vi "Set Collector Speed.vi"(10 "Buttons":T1) -> (3 "Collector Speed":dbl)   [LabVIEW 2011]
uses:
  <vilib>/Rock Robotics/WPI/Joystick/WPI_JoystickButtonState.ctl
  Robot Global Data.vi
panel:
  out "number":u32
  in  "Collector Setting":dbl(slide)=0.6 scale=0.0..1.0
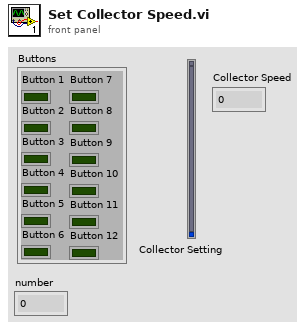
[diagram p1: front panel]
types:
  T1 = typedef "WPI_JoystickButtonState.ctl" = cluster{"Button 1":bool, "Button 2":bool, "Button 3":bool, "Button 4":bool, "Button 5":bool, "Button 6":bool, "Button 7":bool, "Button 8":bool, "Button 9":bool, "Button 10":bool, "Button 11":bool, "Button 12":bool}
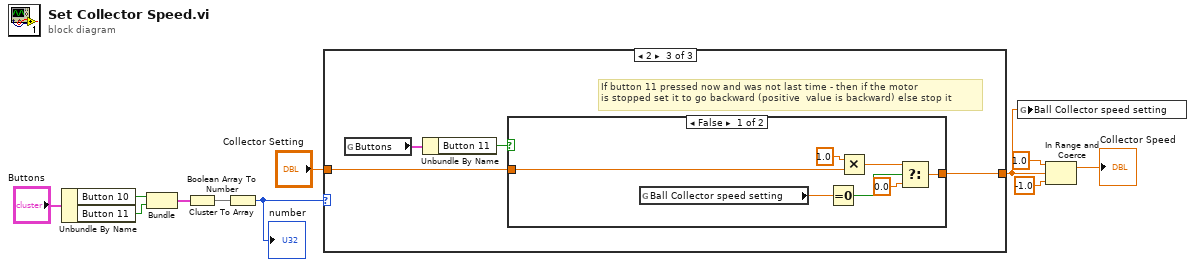
[diagram p0: block diagram]
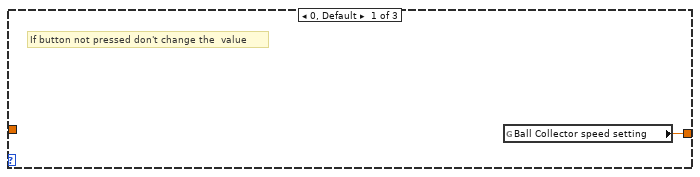
[diagram p2: hidden frame]
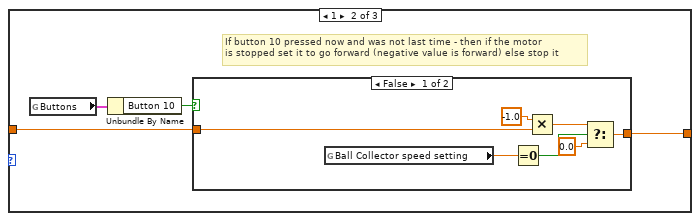
[diagram p3: hidden frame]
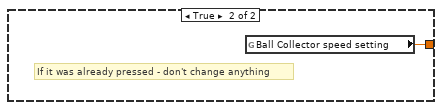
[diagram p4: hidden frame]
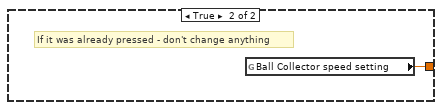
[diagram p5: hidden frame]
diagram:
  n1 = Unbundle By Name("Buttons") -> ("Button 10"=w6:bool, "Button 11"=w5:bool)
  n2 = Bundle("Button 10"=w6, "Button 11"=w5) -> (w4:cluster{"Button 10":bool, "Button 11":bool})  [unwired: 1 in]
  n3 = Cluster To Array(cluster=w4) -> (array=w3:bool[])
  n4 = Boolean Array To Number(Boolean array=w3) -> (number=w2:u32)
  "number" <- w2
  n5 = case shown="2" w2 {
    tunnel: [w12 w14 w26] -> w1
    tunnel: "Collector Setting" -> [_ w13 w25]
    frame 0, Default {
      # "If button not pressed don't change the  value"
      n6 = global read "Robot Global Data.vi" "Ball Collector speed setting"() -> (w12:dbl)
    }
    frame 1 {
      # "If button 10 pressed now and was not last time - then if the motor \nis stopped set it to go forward (negative value is forward) else stop it"
      n7 = global read "Robot Global Data.vi" "Buttons"() -> (w16:T1)
      n8 = Unbundle By Name(w16) -> ("Button 10"=w15:bool)
      n9 = case shown="False" w15 {
        tunnel: [w20 w24] -> w14
        tunnel: w13 -> [w19 _]
        frame False {
          n10 = global read "Robot Global Data.vi" "Ball Collector speed setting"() -> (w22:dbl)
          n11 = Equal To 0?(x=w22) -> (x = 0?=w23:bool)
          n12 = Multiply(x=-1.0, y=w19) -> (x*y=w17:dbl)
          n13 = Select(t=w17, s=w23, f=0.0) -> (s? t:f=w20:dbl)
        }
        frame True {
          # "If it was already pressed - don't change anything"
          n14 = global read "Robot Global Data.vi" "Ball Collector speed setting"() -> (w24:dbl)
        }
      }
    }
    frame 2 {
      # "If button 11 pressed now and was not last time - then if the motor \nis stopped set it to go backward (positive  value is backward) else stop it"
      n15 = global read "Robot Global Data.vi" "Buttons"() -> (w28:T1)
      n16 = Unbundle By Name(w28) -> ("Button 11"=w27:bool)
      n17 = case shown="False" w27 {
        tunnel: [w32 w36] -> w26
        tunnel: w25 -> [w31 _]
        frame False {
          n18 = global read "Robot Global Data.vi" "Ball Collector speed setting"() -> (w34:dbl)
          n19 = Equal To 0?(x=w34) -> (x = 0?=w35:bool)
          n20 = Multiply(x=1.0, y=w31) -> (x*y=w29:dbl)
          n21 = Select(t=w29, s=w35, f=0.0) -> (s? t:f=w32:dbl)
        }
        frame True {
          # "If it was already pressed - don't change anything"
          n22 = global read "Robot Global Data.vi" "Ball Collector speed setting"() -> (w36:dbl)
        }
      }
    }
  }
  n23 = global write "Robot Global Data.vi" "Ball Collector speed setting"(w1) -> ()
  n24 = In Range and Coerce(upper limit=1.0, x=w1, lower limit=-1.0) -> (coerced(x)=→"Collector Speed":dbl)  [unwired: 1 out]
